vi "Read Element of Opened SMOs.vi"(8 "error in (no error)":errorcluster, 10 "index":i32, 11 "Test.Maui 2.0.Panels in":refnum<class "Test.Maui 2.0.Panels.lvclass">) -> (0 "error out":errorcluster, 2 "SMO.lvclass":refnum<class "SMO.lvclass">, 3 "Test.Maui 2.0.Panels out":refnum<class "Test.Maui 2.0.Panels.lvclass">)   [LabVIEW 2020, in "Test.Maui 2.0.Panels.lvclass"]
uses:
  Test.Maui 2.0.Panels.lvclass
  <vilib>/JKI/JKI SMO/SMO/SMO.lvclass
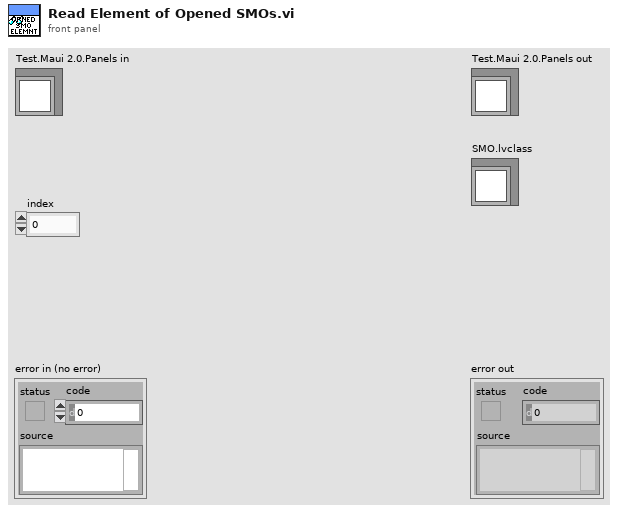
[diagram p1: front panel]
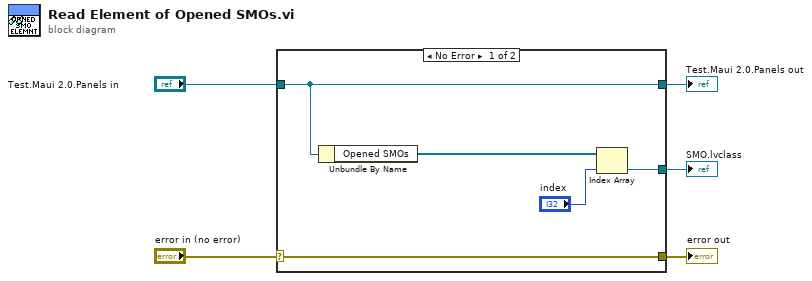
[diagram p0: block diagram]
diagram:
  n1 = case shown="No Error" "error in (no error)" {
    selector: "error in (no error)" -> [w10 w11]
    tunnel: [w10 w11] -> w4
    tunnel: [w9 w12] -> w2
    tunnel: "Test.Maui 2.0.Panels in" -> [w9 w12]
    tunnel: [w6 _] -> w1
    frame No Error {
      n2 = Unbundle By Name(w9) -> ("Opened SMOs"=w8:refnum<class "SMO.lvclass">[])
      n3 = Index Array(array=w8, index="index") -> (element=w6:refnum<class "SMO.lvclass">)
    }
    frame Error {
    }
  }
  "error out" <- w4
  "Test.Maui 2.0.Panels out" <- w2
  "SMO.lvclass" <- w1
